vi "Set Multitone Attributes.vi"(10 "multitone info":T1(array[cluster]), 11 "Display State Attributes in":variant) -> (2 "name":string, 3 "Display State Attributes out":variant)   [LabVIEW 2017, in "Test Signal Configuration.xctl"]
uses:
  <vilib>/addons/_XControls/Function Generator Configuration/Test Signal Configuration.xctl
panel:
  in  "error in (no error)":errorcluster
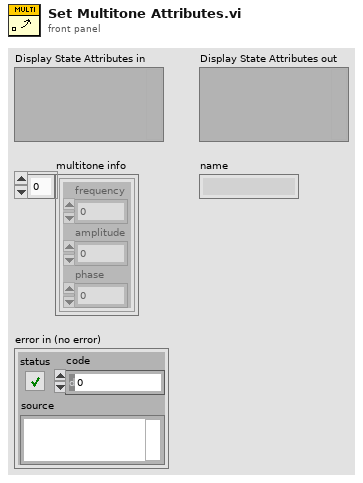
[diagram p1: front panel]
types:
  T1 = cluster{"frequency":dbl, "amplitude":dbl, "phase":dbl}[]
  T2 = typedef "Test Signal Configuration.xctl/signal type.ctl" = enum32{"None", "Tone", "Multitone", "Discrete Sweep", "Continuous Sweep", "Noise"}
  T3 = cluster{"Signal":cluster{"Sample Rate":cluster{"name":string, "default":dbl}, "Signal Type":cluster{"name":string, "signal type":T2}, "Amplitude":cluster{"name":string, "default":dbl}, "Offset":cluster{"name":string, "default":dbl}}, "Function":cluster{"Info":cluster{"name":string, "default":variant}, "Type":cluster{"name":string, "default":u16}, "Frequency":cluster{"name":string, "default":dbl}, "Phase":cluster{"name":string, "default":dbl}}, "Continuous Sweep":cluster{"Info":cluster{"name":string, "default":variant}, "Start":cluster{"name":string, "default":dbl}, "Stop":cluster{"name":string, "default":dbl}, "Duration":cluster{"name":string, "default":dbl}, "Profile":cluster{"name":string, "default":enum16{"Linear", "Logarithmic"}}}, "Discrete Sweep":cluster{"Info":cluster{"name":string, "default":variant}, "Start":cluster{"name":string, "default":dbl}, "Stop":cluster{"name":string, "default":dbl}, "Cycles":cluster{"name":string, "default":dbl}, "Time":cluster{"name":string, "default":dbl}, "Spacing":cluster{"name":string, "default":enum16{"Linear", "Logarithmic"}}, "Steps":cluster{"name":string, "default":i32}}, "Multitone":cluster{"Info":cluster{"name":string, "multitone info":cluster{"frequency":dbl, "amplitude":dbl, "phase":dbl}[]}}, "Noise":cluster{"Info":cluster{"name":string, "default":variant}, "Type":cluster{"name":string, "default":u16}, "Amplitude PDF":cluster{"name":string, "default":enum16{"Gaussian", "Rectangular", "Triangular"}}, "Level":cluster{"name":string, "default":dbl}, "Seed":cluster{"name":string, "default":i32}}, "Configuration":cluster{"Min Frequency":cluster{"name":string, "default":dbl}, "Max Frequency":cluster{"name":string, "default":dbl}, "Max Amplitude":cluster{"name":string, "default":dbl}}}
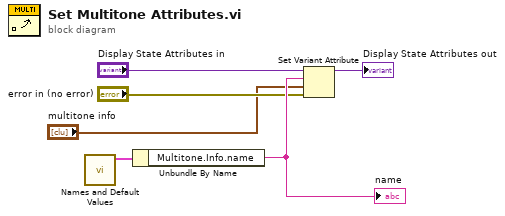
[diagram p0: block diagram]
diagram:
  n1 = call <vilib>:"Names and Default Values.vi"() -> ("Names and Default Values"=w5:T3)  [unwired: 11 in]
  n2 = Unbundle By Name(w5) -> ("Multitone.Info.name"=w6:string)
  "name" <- w6
  n3 = Set Variant Attribute(Variant="Display State Attributes in", name=w6, value="multitone info", error in="error in (no error)") -> (Variant out=→"Display State Attributes out":variant)  [unwired: 2 out]
